vi "fgv_PotentialField_config.vi"(7 "cmd":T2, 11 "pf-val":T1) -> (3 "pf-val out":T1)   [LabVIEW 2019]
uses:
  Ctrl/cmd_common.ctl
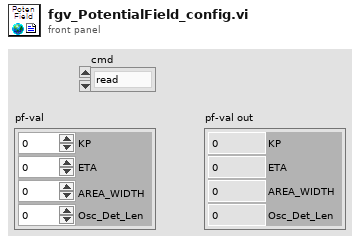
[diagram p1: front panel]
types:
  T1 = cluster{"KP":dbl, "ETA":dbl, "AREA_WIDTH":dbl, "Osc_Det_Len":u32}
  T2 = typedef "cmd_common.ctl" = enum16{"read", "write"}
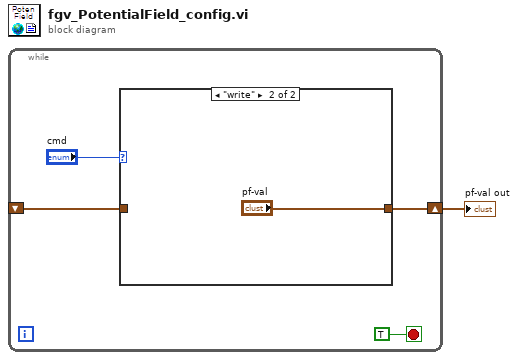
[diagram p0: block diagram]
diagram:
  n1 = while {
    shift-right: [w3] -> w1
    shift-left: _ -> [w2]
    stop <- TRUE stop-if-true
    n2 = case shown="\"write\"" "cmd" {
      tunnel: [w6 "pf-val"] -> w3
      tunnel: w2 -> [w6 _]
      frame "read", Default {
      }
      frame "write" {
      }
    }
  }
  "pf-val out" <- w1
